vi "Welcome Message (SubVI).vi"() -> (0 "String":string)   [LabVIEW 2019]
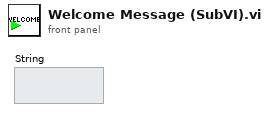
[diagram p1: front panel]
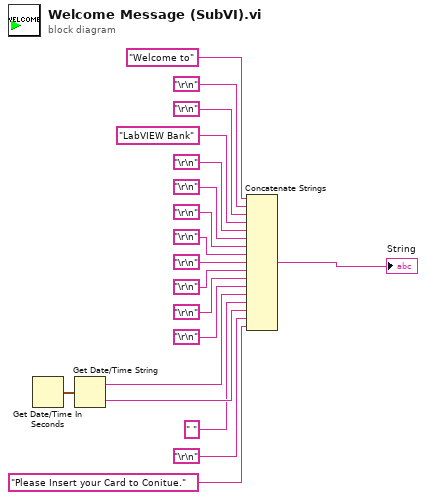
[diagram p0: block diagram]
diagram:
  n1 = Get Date/Time In Seconds() -> (seconds since 1Jan1904=w1:timestamp)
  n2 = Get Date/Time String(seconds (now)=w1) -> (date string=w16:string, time string=w15:string)  [unwired: 2 in]
  n3 = Concatenate Strings("Welcome to" ("string"), "\r\n", "\r\n", "LabVIEW Bank" ("string"), "\r\n", "\r\n", "\r\n", "\r\n", "\r\n", "\r\n", "\r\n", "\r\n", w16, " ", w15, "\r\n", "Please Insert your Card to Conitue." ("string")) -> (→"String":string)
